vi "Generate Date.vi"() -> (3 "chaîne de date/heure":string)   [LabVIEW 2020, in "Library Commun.lvlib"]
uses:
  Library Commun.lvlib
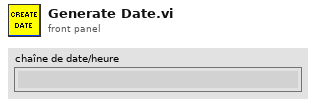
[diagram p1: front panel]
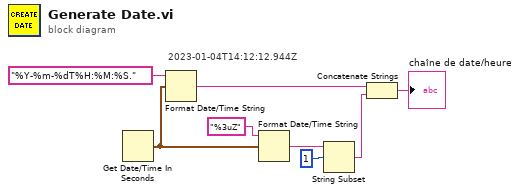
[diagram p0: block diagram]
diagram:
  # "2023-01-04T14:12:12.944Z"
  n1 = Get Date/Time In Seconds() -> (seconds since 1Jan1904=w6:timestamp)
  n2 = Format Date/Time String(time format string (%c)="%Y-%m-%dT%H:%M:%S." ("chaîne de format de l'heure (%c)"), seconds (now)=w6) -> (date/time string=w5:string)  [unwired: 1 in]
  n3 = Format Date/Time String(time format string (%c)="%3uZ" ("chaîne de format de l'heure (%c)"), seconds (now)=w6) -> (date/time string=w4:string)  [unwired: 1 in]
  n4 = String Subset(string=w4, offset (0)=1) -> (substring=w2:string)  [unwired: 1 in]
  n5 = Concatenate Strings(w5, w2) -> (→"chaîne de date/heure":string)
